vi "Hide Controls.vi"(6 "Variant in":variant, 7 "Shift Pressed?":bool, 8 "error in (no error)":errorcluster, 10 "QD Combo Box Ref":refnum<vi>, 11 "QD Launch VI Ref":refnum<vi>) -> (0 "error out":errorcluster, 4 "Variant out":variant)   [LabVIEW 2020, in "Control Operation.lvlib"]
doc: "Hide Controls"
uses:
  Control Operation.lvlib
panel:
  in  "Undo Name":string="Hide Controls"
  # "Do not change the connector pane of this VI.\n\nSee the block diagram for directions on how to use this template."
  # "Specify the name of the Undo transaction"
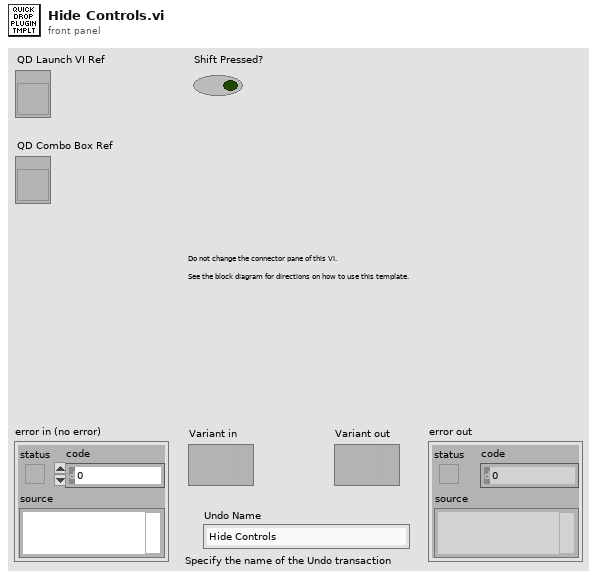
[diagram p1: front panel]
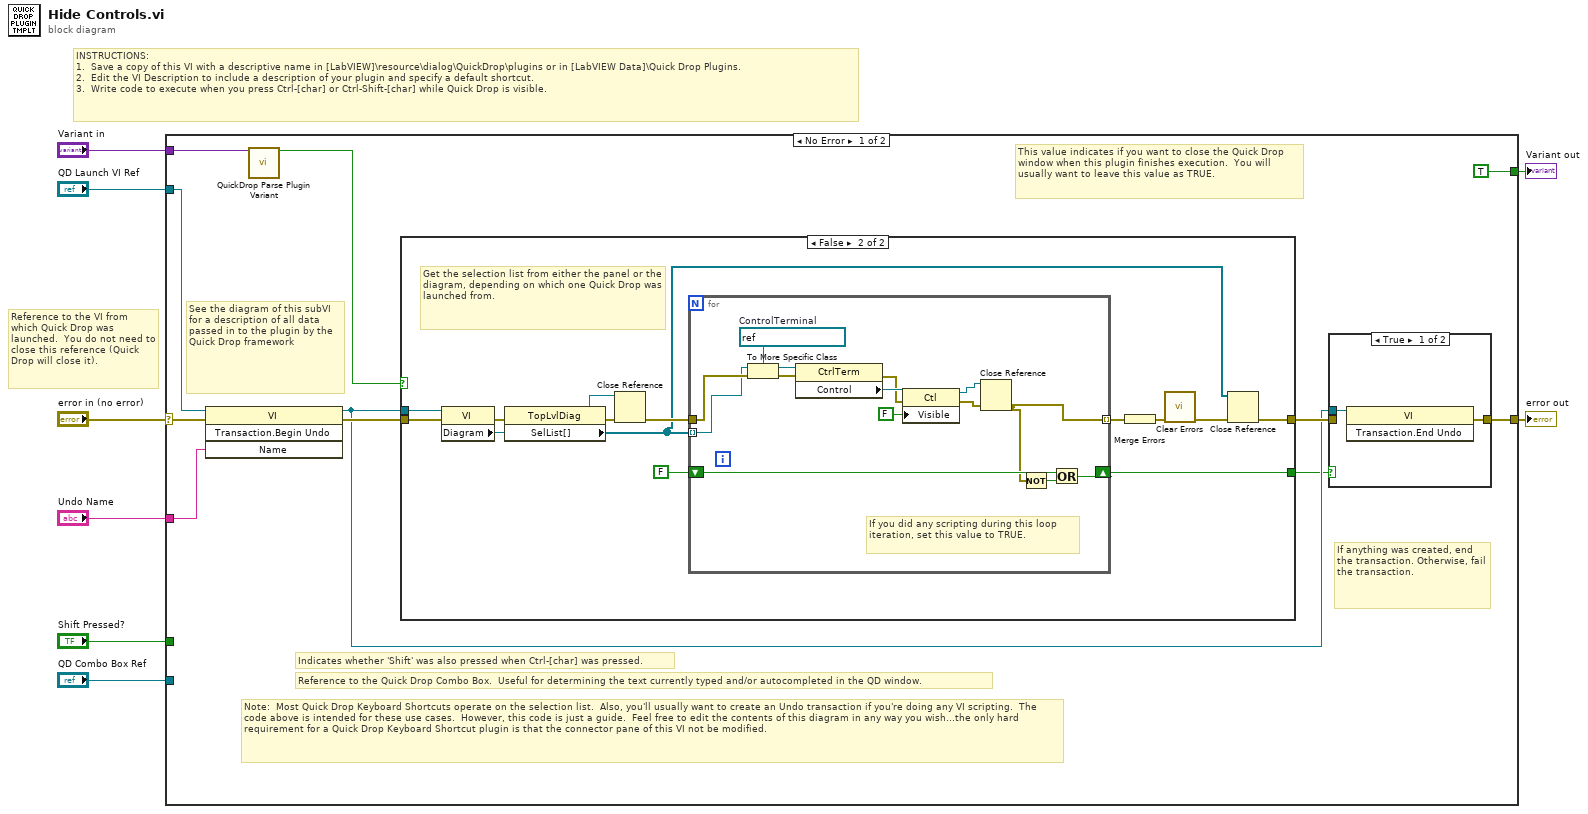
[diagram p0: block diagram]
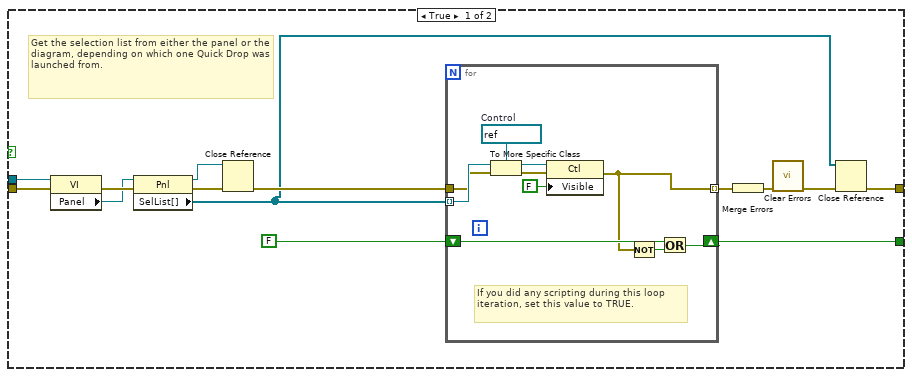
[diagram p2: hidden frame]
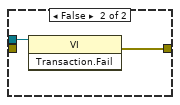
[diagram p3: hidden frame]
diagram:
  # "Reference to the VI from which Quick Drop was launched.  You do not need to close this reference (Quick Drop will close it)."
  # "INSTRUCTIONS:\n1.  Save a copy of this VI with a descriptive name in [LabVIEW]\\resource\\dialog\\QuickDrop\\plugins or in [LabVIEW Data]\\Quick Drop Plugins.\n2.  Edit the VI Description to include a description of your plugin and specify a default shortcut. \n3.  Write code to execute when you press Ctrl-[char] or Ctrl-Shift-[char] while Quick Drop is visible."
  n1 = case shown="No Error" "error in (no error)" {
    selector: "error in (no error)" -> [w18 w76]
    tunnel: [w12 w76] -> w7
    tunnel: "QD Launch VI Ref" -> [w17 _]
    tunnel: "Shift Pressed?" -> [_ _]
    tunnel: "QD Combo Box Ref" -> [_ _]
    tunnel: "Variant in" -> [w19 _]
    tunnel: "Undo Name" -> [w16 _]
    tunnel: [TRUE _] -> w1
    frame No Error {
      # "Note:  Most Quick Drop Keyboard Shortcuts operate on the selection list.  Also, you'll usually want to create an Undo transaction if you're doing any VI scripting.  The code above is intended for these use cases.  However, this code is just a guide.  Feel free to edit the contents of this diagram in any way you wish...the only hard requirement for a Quick Drop Keyboard Shortcut plugin is that the connector pane of this VI not be modified."
      # "If anything was created, end the transaction. Otherwise, fail the transaction."
      # "This value indicates if you want to close the Quick Drop window when this plugin finishes execution.  You will usually want to leave this value as TRUE."
      # "See the diagram of this subVI for a description of all data passed in to the plugin by the Quick Drop framework"
      # "Reference to the Quick Drop Combo Box.  Useful for determining the text currently typed and/or autocompleted in the QD window."
      # "Indicates whether 'Shift' was also pressed when Ctrl-[char] was pressed."
      n2 = invoke class="VI" method="Transaction.Begin Undo"(reference=w17, error in=w18, "Name"=w16) -> (reference out=w10:refnum<vi>, error out=w13:errorcluster)  [unwired: 1 in, 2 out]
      n3 = call <vilib>:"QuickDrop Parse Plugin Variant.vi"("QDKS Variant in"=w19) -> ("QD Launch VI Panel?"=w14:bool)  [unwired: 12 in, 2 out]
      n4 = case shown="False" w14 {
        tunnel: w13 -> [w33 w57]
        tunnel: [w23 w47] -> w11
        tunnel: w10 -> [w31 w55]
        tunnel: [w29 w53] -> w9
        frame True {
          # "Get the selection list from either the panel or the diagram, depending on which one Quick Drop was launched from."
          n5 = property class="VI"(reference=w31, error in=w33) -> (error out=w28:errorcluster, "Panel"=w27:refnum<vi>)  [unwired: 1 out]
          n6 = property class="Pnl"(reference=w27, error in=w28) -> (reference out=w25:refnum<vi>, error out=w26:errorcluster, "SelList[]"=w22:refnum<vi>[])
          n7 = Close Reference(reference=w25, error in (no error)=w26) -> (error out=w32:errorcluster)
          n8 = for {
            shift-right: [w42] -> w29
            shift-left: FALSE -> [w43]
            tunnel: w22 -> [w41] mode=indexing
            tunnel: w32 -> [w38]
            tunnel: [w36] -> w24 mode=indexing
            w37 = refnum<vi> refnum  # Control
            # "If you did any scripting during this loop iteration, set this value to TRUE."
            n9 = To More Specific Class(target class=w37, reference=w41, error in=w38) -> (specific class reference=w40:refnum<vi>, error out=w39:errorcluster)
            n10 = property class="Ctl"(reference=w40, error in=w39, "Visible"=FALSE) -> (error out=w36:errorcluster)  [unwired: 1 out]
            n11 = Not(x=w36) -> (.not. x?=w35:bool)
            n12 = Or(x=w43, y=w35) -> (x .or. y?=w42:bool)
          }
          n13 = Merge Errors(w24) -> (w20:errorcluster)
          n14 = call <vilib>:"Clear Errors.vi"("error in (no error)"=w20) -> ("error out"=w21:errorcluster)  [unwired: 5 in, 1 out]
          n15 = Close Reference(reference=w22, error in (no error)=w21) -> (error out=w23:errorcluster)
        }
        frame False {
          # "Get the selection list from either the panel or the diagram, depending on which one Quick Drop was launched from."
          n16 = property class="VI"(reference=w55, error in=w57) -> (error out=w52:errorcluster, "Diagram"=w51:refnum<vi>)  [unwired: 1 out]
          n17 = property class="TopLvlDiag"(reference=w51, error in=w52) -> (reference out=w49:refnum<vi>, error out=w50:errorcluster, "SelList[]"=w46:refnum<vi>[])
          n18 = Close Reference(reference=w49, error in (no error)=w50) -> (error out=w56:errorcluster)
          n19 = for {
            shift-right: [w70] -> w53
            shift-left: FALSE -> [w71]
            tunnel: w46 -> [w59] mode=indexing
            tunnel: w56 -> [w60]
            tunnel: [w58] -> w48 mode=indexing
            w66 = refnum<vi> refnum  # ControlTerminal
            # "If you did any scripting during this loop iteration, set this value to TRUE."
            n20 = To More Specific Class(target class=w66, reference=w59, error in=w60) -> (specific class reference=w68:refnum<vi>, error out=w67:errorcluster)
            n21 = property class="CtrlTerm"(reference=w68, error in=w67) -> (error out=w61:errorcluster, "Control"=w65:refnum<vi>)  [unwired: 1 out]
            n22 = property class="Ctl"(reference=w65, error in=w61, "Visible"=FALSE) -> (reference out=w62:refnum<vi>, error out=w63:errorcluster)
            n23 = Close Reference(reference=w62, error in (no error)=w63) -> (error out=w58:errorcluster)
            n24 = Not(x=w58) -> (.not. x?=w69:bool)
            n25 = Or(x=w71, y=w69) -> (x .or. y?=w70:bool)
          }
          n26 = Merge Errors(w48) -> (w44:errorcluster)
          n27 = call <vilib>:"Clear Errors.vi"("error in (no error)"=w44) -> ("error out"=w45:errorcluster)  [unwired: 5 in, 1 out]
          n28 = Close Reference(reference=w46, error in (no error)=w45) -> (error out=w47:errorcluster)
        }
      }
      n29 = case shown="True" w9 {
        tunnel: w10 -> [w72 w74]
        tunnel: [w73 w75] -> w12
        tunnel: w11 -> [_ _]
        frame True {
          n30 = invoke class="VI" method="Transaction.End Undo"(reference=w72) -> (error out=w73:errorcluster)  [unwired: 2 in, 2 out]
        }
        frame False {
          n31 = invoke class="VI" method="Transaction.Fail"(reference=w74) -> (error out=w75:errorcluster)  [unwired: 2 in, 2 out]
        }
      }
    }
    frame Error {
    }
  }
  "error out" <- w7
  "Variant out" <- w1
